vi "O3 49i Serial Test.vi"() -> ()   [LabVIEW 2014]
uses:
  <vilib>/Instr/_visa.llb/VISA Set IO Buffer Mask.ctl
  <vilib>/Instr/_visa.llb/VISA Configure Serial Port (Instr).vi
panel:
  in  "VISA resource name 2":refnum<visa-resource-name>="ASRL6::INSTR"
  out "Loop count":i32
  out "runninig?":bool
  out "error out":errorcluster
  out "Data Out":string
  out "Max Acq Time":u32
  out "Waveform Chart":u32(graph)
  in  "milliseconds to wait":u32=330
  in  "ID":string="»"
  out "Command In":string
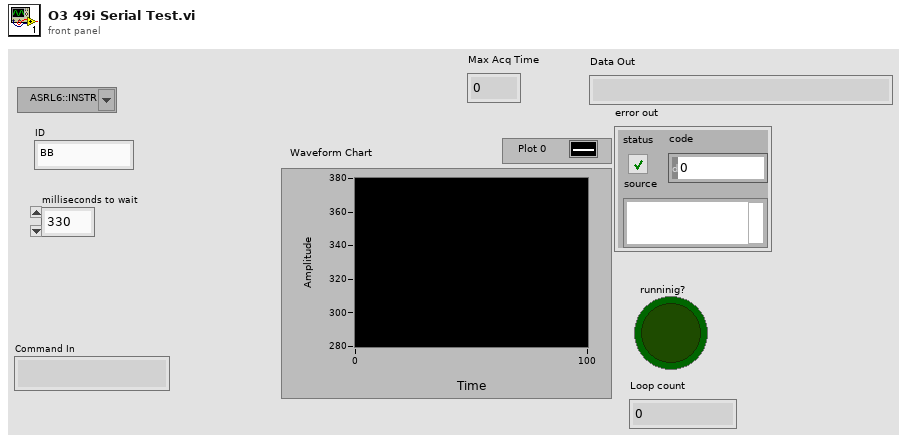
[diagram p1: front panel]
types:
  T1 = typedef "VISA Set IO Buffer Mask.ctl" = u16
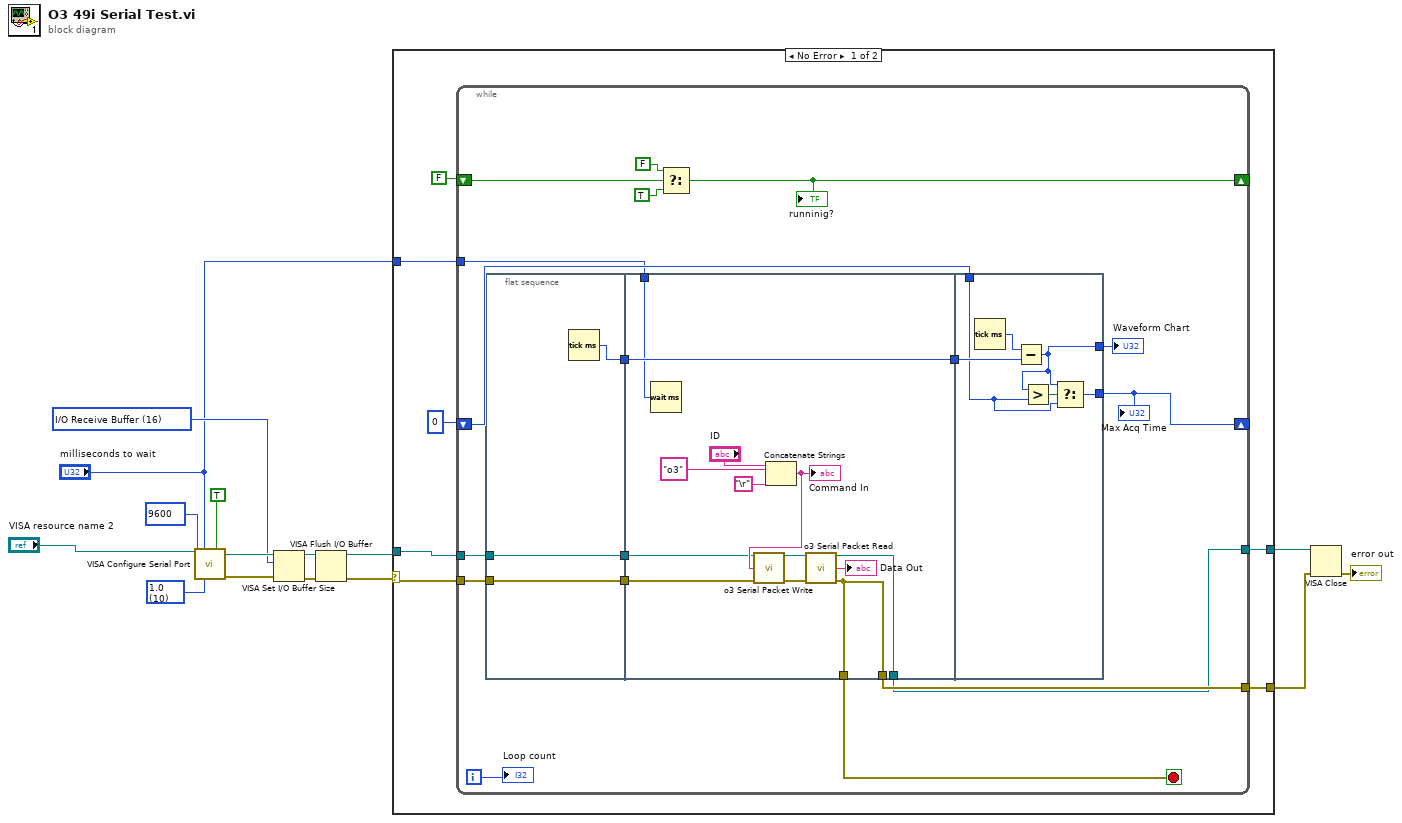
[diagram p0: block diagram]
diagram:
  w4 = u16 10 items=["1.0"=10, "1.5"=15, "2.0"=20] ("stop bits (10: 1 bit)")
  w7 = T1 16 items=["I/O Receive Buffer"=16, "I/O Transmit Buffer"=32, "I/O Receive and Transmit Buffer"=48] ("Mask")
  n1 = call-poly "VISA Configure Serial Port"("VISA resource name"="VISA resource name 2", "timeout (10sec)"="milliseconds to wait", "Enable Termination\nChar (T)"=TRUE ("Enable Termination\nChar (T)"), "baud rate (9600)"=u32 9600, "stop bits (10: 1 bit)"=w4) -> ("VISA resource name out"=w10:refnum<visa-resource-name>, "error out"=w11:errorcluster)  [unwired: 9 in]
  n2 = VISA Set I/O Buffer Size(VISA resource name=w10, mask (16)=w7, error in (no error)=w11) -> (VISA resource name out=w6:refnum<visa-resource-name>, error out=w12:errorcluster)  [unwired: 1 in]
  n3 = VISA Flush I/O Buffer(VISA resource name=w6, error in (no error)=w12) -> (VISA resource name out=w9:refnum<visa-resource-name>, error out=w8:errorcluster)  [unwired: 1 in]
  n4 = case shown="No Error" w8 {
    selector: w8 -> [w20 w63]
    tunnel: w9 -> [w22 w64]
    tunnel: [w19 w63] -> w15
    tunnel: [w18 w64] -> w14
    tunnel: "milliseconds to wait" -> [w17 _]
    frame No Error {
      n5 = while {
        tunnel: w22 -> [w36]
        tunnel: w20 -> [w35]
        shift-right: [w33] -> _
        shift-left: 0 -> [w34]
        tunnel: [w30] -> w19
        tunnel: [w29] -> w18
        tunnel: w17 -> [w28]
        shift-right: [w24] -> _
        shift-left: FALSE -> [w27]
        i -> [w23]
        stop <- w31 stop-if-true
        n6 = flat-sequence {
          tunnel: w35 -> [w42]
          tunnel: w36 -> [w43]
          tunnel: [w43] -> w40
          tunnel: [w42] -> w39
          tunnel: [w41] -> w38
          tunnel: w40 -> [w50]
          tunnel: w39 -> [w49]
          tunnel: [w48] -> w37
          tunnel: w38 -> [w48]
          tunnel: [w46] -> w31
          tunnel: [w46] -> w30
          tunnel: [w45] -> w29
          tunnel: w28 -> [w44]
          tunnel: w37 -> [w61]
          tunnel: w34 -> [w59]
          tunnel: [w58] -> w33
          tunnel: [w57] -> w32
          frame #0 {
            n7 = Tick Count (ms)() -> (millisecond timer value=w41:u32)
          }
          frame #1 {
            n8 = Wait (ms)(milliseconds to wait=w44) -> ()  [unwired: 1 out]
            n9 = Concatenate Strings("ID", "o3" ("string"), "\r") -> (w52:string)
            "Command In" <- w52
            n10 = call "o3 Serial Packet Write.vi"("VISA resource name In"=w50, "Data in"=w52, "error in (no error)"=w49) -> ("VISA resource name Out"=w55:refnum<visa-resource-name>, "error out"=w54:errorcluster)  [unwired: 11 in]
            n11 = call "o3 Serial Packet Read.vi"("VISA resource In"=w55, "error in"=w54) -> ("VISA resource Out"=w45:refnum<visa-resource-name>, "Data Out"=→"Data Out":string, "error out"=w46:errorcluster)  [unwired: 11 in]
          }
          frame #2 {
            n12 = Tick Count (ms)() -> (millisecond timer value=w62:u32)
            n13 = Subtract(x=w62, y=w61) -> (x-y=w57:u32)
            n14 = Greater?(x=w57, y=w59) -> (0:w60:bool)
            n15 = Select(t=w57, s=w60, f=w59) -> (s? t:f=w58:u32)
          }
        }
        n16 = Select(t=FALSE, s=w27, f=TRUE) -> (s? t:f=w24:bool)
        "runninig?" <- w24
        "Waveform Chart" <- w32
        "Max Acq Time" <- w33
        "Loop count" <- w23
      }
    }
    frame Error {
    }
  }
  n17 = VISA Close(VISA resource name=w14, error in (no error)=w15) -> (error out=→"error out":errorcluster)
